vi "Input Kinds.vi"(8 "error in (no error)":errorcluster, 11 "RGetInputKindList in":refnum<class "RGetInputKindList.lvclass">) -> (0 "error out":errorcluster, 2 "Input Kinds":string[](array[string]), 3 "RGetInputKindList out":refnum<class "RGetInputKindList.lvclass">)   [LabVIEW 2020, in "obs-websocket.lvlib" / "RGetInputKindList.lvclass"]
uses:
  RGetInputKindList.lvclass
  RGetInputKindList.lvclass/RGetInputKindList.ctl
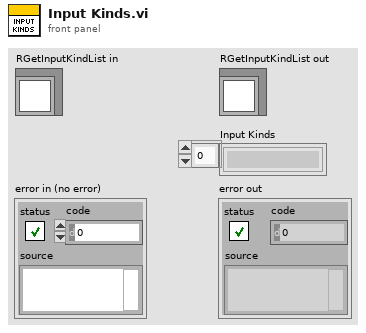
[diagram p1: front panel]
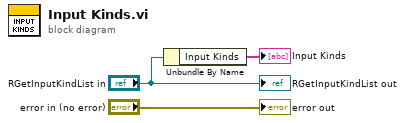
[diagram p0: block diagram]
diagram:
  n1 = Unbundle By Name("RGetInputKindList in") -> ("Input Kinds"=→"Input Kinds":string[])
  "error out" <- "error in (no error)"
  "RGetInputKindList out" <- "RGetInputKindList in"
